vi "audio_processor.vi"(8 "error in (no error)":errorcluster) -> (0 "error out":errorcluster)   [LabVIEW 2020]
uses:
  FGVs/FGVstates.ctl
  <vilib>/sound2/lvsound2.llb/Sound Output Write (DBL).vi
panel:
  out "data":waveform(dbl)[](array[waveform])
  out "Execution time loop":u32
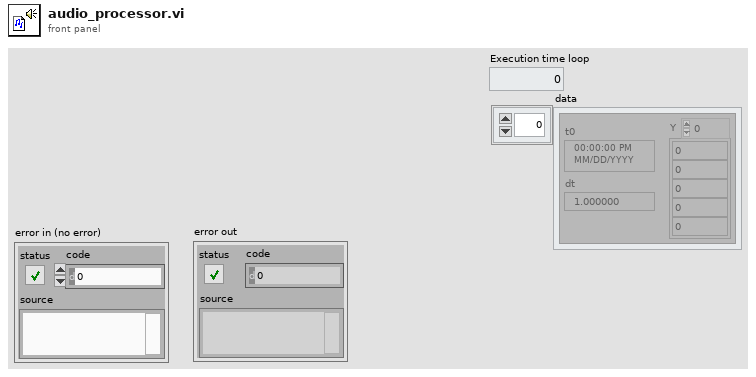
[diagram p1: front panel]
types:
  T1 = typedef "FGVstates.ctl" = enum16{"Init", "Set", "Get", "De-Init"}
  T2 = typedef "data_exchange_fgv.ctl" = cluster{"queue states":refnum<queue>, "audio data":refnum<queue>, "error queue":refnum<queue>}
  T3 = typedef "Sound Output Task ID.ctl" = u32
  T4 = typedef "AppStates.ctl" = enum16{"Init", "Scan Music Dir", "Idle", "Playback", "Enqueue samples", "Pause playback", "Stop playback", "Exit"}
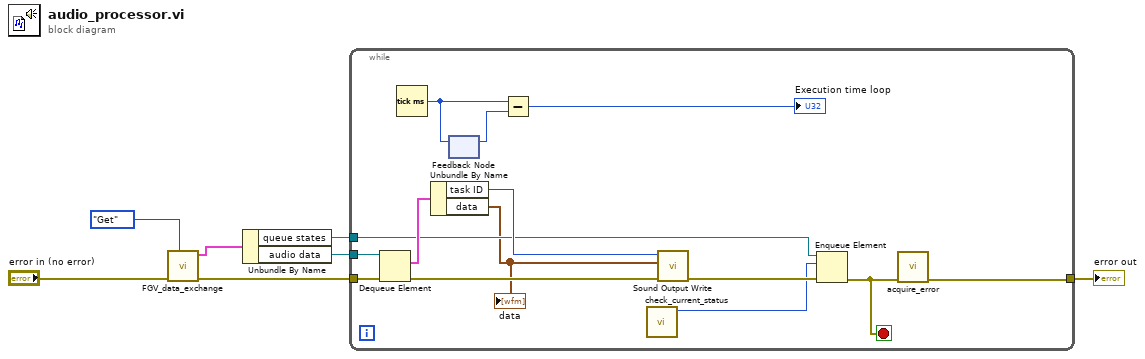
[diagram p0: block diagram]
diagram:
  n1 = call "FGV_data_exchange.vi"("FGV states"=FGVstates."Get", "error in (no error)"="error in (no error)") -> ("error out"=w4:errorcluster, "main_cycle_queue"=w3:T2)  [unwired: 8 in]
  n2 = Unbundle By Name(w3) -> ("queue states"=w1:refnum<queue>, "audio data"=w2:refnum<queue>)
  n3 = while {
    tunnel: w4 -> [w17]
    tunnel: [w13] -> w7
    tunnel: w2 -> [w21]
    tunnel: w1 -> [w15]
    stop <- w12 stop-if-true
    n4 = Dequeue Element(queue=w21, error in (no error)=w17) -> (element=w20:cluster{"task ID":T3, "data":waveform(dbl)[]}, error out=w14:errorcluster)  [unwired: 1 in, 2 out]
    n5 = Tick Count (ms)() -> (millisecond timer value=w9:u32)
    n6 = Unbundle By Name(w20) -> ("task ID"=w19:T3, "data"=w8:waveform(dbl)[])
    "data" <- w8
    n7 = feedback-in #1(w9) -> ()
    n8 = feedback #1() -> (w10:u32)  [unwired: 1 in]
    n9 = Subtract(x=w9, y=w10) -> (x-y=→"Execution time loop":u32)
    n10 = call "check_current_status.vi"() -> ("operation to enqueue"=w16:T4)  [unwired: 10 in, 1 out]
    n11 = call-poly <vilib>:"Sound Output Write.vi"("error in (no error)"=w14, "data"=w8, "task ID"=w19) -> ("error out"=w18:errorcluster)  [unwired: 7 in, 1 out]
    n12 = Enqueue Element(queue=w15, element=w16, error in (no error)=w18) -> (error out=w12:errorcluster)  [unwired: 1 in, 2 out]
    n13 = call "acquire_error.vi"("error in (no error)"=w12) -> ("error out"=w13:errorcluster)  [unwired: 10 in]
  }
  "error out" <- w7
